vi "Filter Available Channels.vi"(11 "DAQmx Shortcuts":T1[](array[typedef])) -> (2 "DAQmx DI Shortcuts":T1[](array[typedef]), 3 "DAQmx AI Shortcuts":T1[](array[typedef]))   [LabVIEW 2019, in "DAQmx.lvlib"]
doc: "Filter all possible DAQmx events down to the global channels configured in MAX."
uses:
  DAQmx.lvlib
  DAQmx Shortcut.ctl
  <resource>/objmgr/daqmx.rc
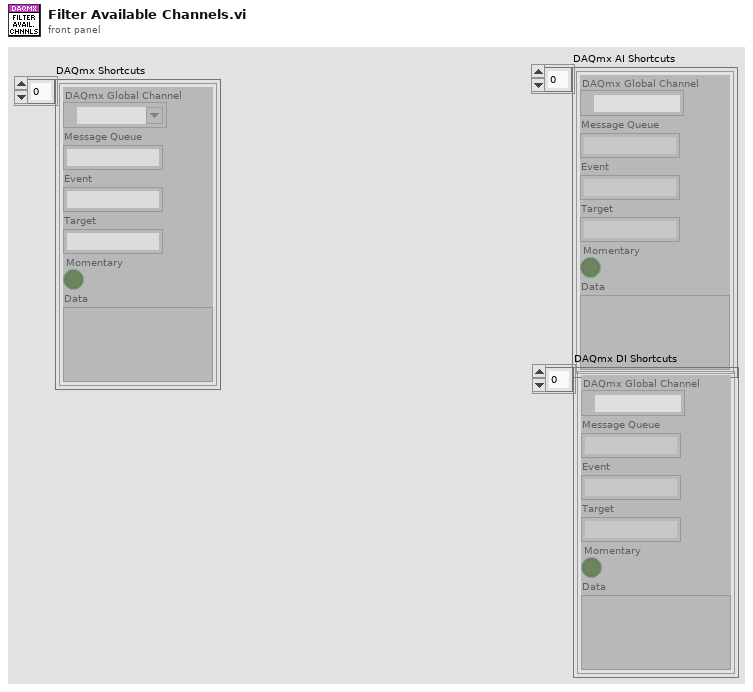
[diagram p1: front panel]
types:
  T1 = typedef "DAQmx.lvlib/DAQmx Shortcut.ctl" = cluster{"DAQmx Global Channel":refnum<k21>, "Message Queue":string, "Event":string, "Target":string, "Momentary":bool, "Data":variant}
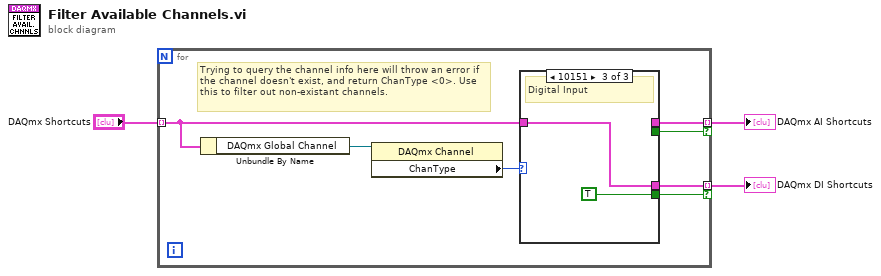
[diagram p0: block diagram]
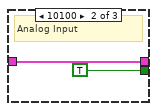
[diagram p3: hidden frame]
diagram:
  n1 = for {
    tunnel: "DAQmx Shortcuts" -> [w8] mode=indexing
    tunnel: [w7] -> w2 mode=indexing if=w5
    tunnel: [w6] -> w1 mode=indexing if=w4
    # "Trying to query the channel info here will throw an error if the channel doesn't exist, and return ChanType <0>. Use this to filter out non-existant channels."
    n2 = Unbundle By Name(w8) -> ("DAQmx Global Channel"=w10:refnum<k21>)
    n3 = property class="DAQmx Channel"(reference=w10) -> ("ChanType"=w9:i32)  [unwired: 1 in, 2 out]
    n4 = case shown="10151" w9 {
      tunnel: w8 -> [_ w12 w14]
      tunnel: [_ w12 _] -> w7
      tunnel: [_ TRUE _] -> w5
      tunnel: [_ _ w14] -> w6
      tunnel: [_ _ TRUE] -> w4
      frame Default {
      }
      frame 10100 {
        # "Analog Input"
      }
      frame 10151 {
        # "Digital Input"
      }
    }
  }
  "DAQmx AI Shortcuts" <- w2
  "DAQmx DI Shortcuts" <- w1
